vi "Read PINGRESP.vi"(8 "error in (no error)":errorcluster, 11 "connection ID":refnum<k5>) -> (0 "error out":errorcluster, 2 "PingResp Message":u8[](array[numeric]) format="%x", 3 "connection ID out":refnum<k5>)   [LabVIEW 2020, in "DAQIO MQTT.lvlib"]
doc: "This VI responds to a PINREQ message and corresponds to a \"PING\" reply. \n\n© 2015 - daq.io, LLC - Peter Adelhardt"
uses:
  DAQIO MQTT.lvlib
  Controls/MessageType.ctl
  Controls/Retain_Flag.ctl
  Controls/DUP Flag.ctl
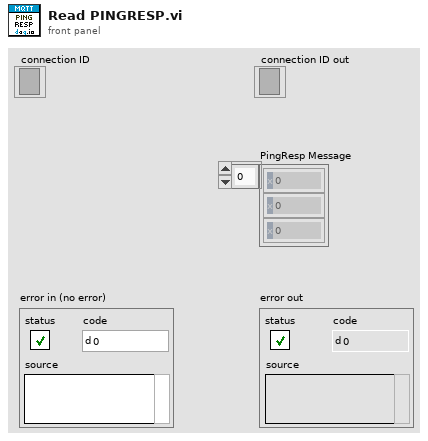
[diagram p1: front panel]
types:
  T1 = typedef "DAQIO MQTT.lvlib/DUP Flag.ctl" = bool
  T2 = enum8{"At most once", "At least once", "Exactly once", "Reserved"}
  T3 = typedef "DAQIO MQTT.lvlib/Retain_Flag.ctl" = bool
  T4 = typedef "DAQIO MQTT.lvlib/MessageType.ctl" = enum32{"Reserved", "CONNECT", "CONNACK", "PUBLISH", "PUBACK", "PUBREC", "PUBREL", "PUBCOMP", "SUBSCRIBE", "SUBACK", "UNSUBSCRIBE", "UNSUBACK", "PINGREQ", "PINGRESP", "DISCONNECT", "Reserved2"}
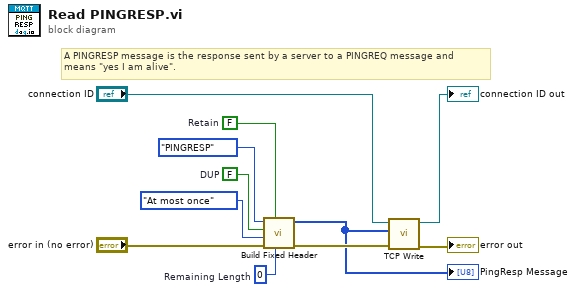
[diagram p0: block diagram]
diagram:
  w6 = u32 0  # Remaining Length
  w8 = T1 FALSE  # DUP
  w10 = T3 FALSE  # Retain
  # "A PINGRESP message is the response sent by a server to a PINGREQ message and\nmeans \"yes I am alive\"."
  n1 = call "Build Fixed Header.vi"("Remaining Length"=w6, "Retain"=w10, "error in (no error)"="error in (no error)", "QoS"=T2."At most once", "DUP"=w8, "MessageType"=MessageType."PINGRESP") -> ("error out"=w5:errorcluster, "Fixed Header"=w1:u8[])  [unwired: 4 in]
  "PingResp Message" <- w1
  n2 = call "TCP Write.vi"("error in (no error)"=w5, "data in"=w1, "connection ID"="connection ID") -> ("error out"=→"error out":errorcluster, "connection ID out"=→"connection ID out":refnum<k5>)  [unwired: 6 in, 1 out]
